vi "save_channel_settings.vi"(8 "error in":errorcluster, 11 "swabian_channel_settings":T1=[{"Threshold (V)"=0.5, "Input Delay (ps)"=0, "Dead Time (ps)"=6000}, {"Threshold (V)"=0.5, "Input Delay (ps)"=0, "Dead Time (ps)"=6000}, {"Threshold (V)"=0.5, "Input Delay (ps)"=0, "Dead Time (ps)"=6000}, {"Threshold (V)"=0.5, "Input Delay (ps)"=0, "Dead Time (ps)"=6000}, {"Threshold (V)"=0.5, "Input Delay (ps)"=0, "Dead Time (ps)"=6000}, {"Threshold (V)"=0.5, "Input Delay (ps)"=0, "Dead Time (ps)"=6000}, {"Threshold (V)"=0.5, "Input Delay (ps)"=0, "Dead Time (ps)"=6000}, {"Threshold (V)"=0.5, "Input Delay (ps)"=0, "Dead Time (ps)"=6000}] {"Dead Time (ps)" min=0 step=6000; "Input Delay (ps)" min=0 step=1; "Threshold (V)" min=0.0 max=2.5 step=0.1}) -> (0 "error out":errorcluster)   [LabVIEW 2018]
uses:
  swabian_channel_settings.ctl
  channel_settings.ctl
  <vilib>/Utility/xml.llb/Write to XML File(string).vi
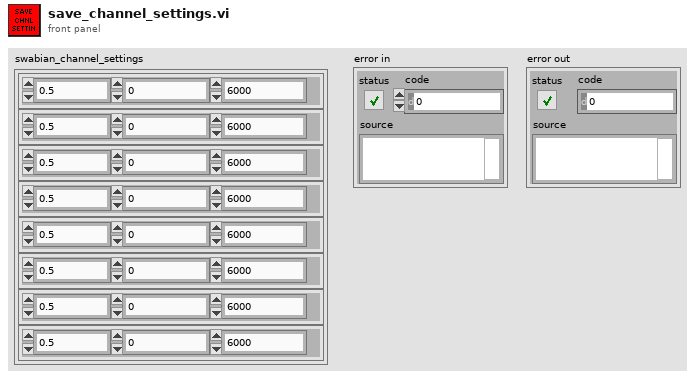
[diagram p1: front panel]
types:
  T1 = typedef "swabian_channel_settings.ctl" = T2[]
  T2 = typedef "channel_settings.ctl" = cluster{"Threshold (V)":dbl, "Input Delay (ps)":i64, "Dead Time (ps)":i64}
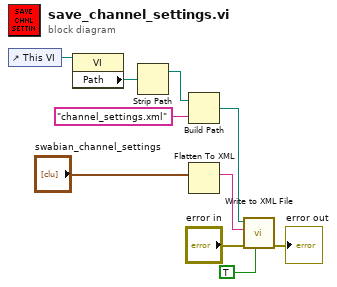
[diagram p0: block diagram]
diagram:
  n1 = control-ref of="This VI"() -> (w10:refnum<vi>)
  n2 = property class="VI"(reference=w10) -> ("Path"=w9:path)  [unwired: 1 in, 2 out]
  n3 = Strip Path(path=w9) -> (stripped path=w8:path)  [unwired: 1 out]
  n4 = Build Path(base path=w8, name or relative path="channel_settings.xml") -> (appended path=w4:path)
  n5 = Flatten To XML(anything="swabian_channel_settings") -> (xml string=w3:string)
  n6 = call-poly <vilib>:"Write to XML File.vi"("Standalone? (T)"=TRUE, "error in (no error)"="error in", "XML Input"=w3, "XML File Path"=w4) -> ("error out"=→"error out":errorcluster)  [unwired: 5 in, 2 out]
